vi "Field Add Test Step Field.vi"(6 "nDataType":T1, 7 "sDisplayName":string, 8 "sUnits":string, 9 "sValue":string, 10 "sxFieldId":string, 11 "Fields In":T2[](array[typedef])) -> (3 "Fields Out":T2[](array[typedef]))   [LabVIEW 2011]
uses:
  Field Record.ctl
  Field DataTypes.ctl
  Field NextItem.ctl
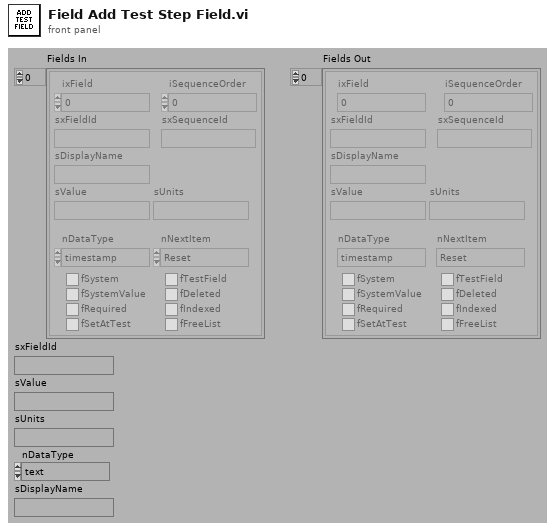
[diagram p1: front panel]
types:
  T1 = typedef "Field DataTypes.ctl" = enum32{"text", "numeric", "list", "timestamp", "boolean"}
  T2 = typedef "Field Record.ctl" = cluster{"ixField":i32, "iSequenceOrder":i32, "sxFieldId":string, "sxSequenceId":string, "sDisplayName":string, "sValue":string, "sUnits":string, "nDataType":T1, "nNextItem":T3, "fSystem":bool, "fSystemValue":bool, "fRequired":bool, "fSetAtTest":bool, "fTestField":bool, "fDeleted":bool, "fIndexed":bool, "fFreeList":bool}
  T3 = typedef "Field NextItem.ctl" = enum32{"Reset", "Retain", "Auto-Increment"}
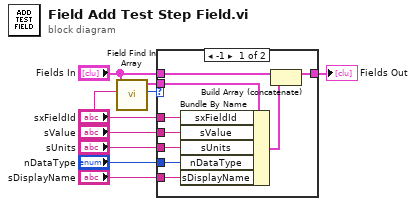
[diagram p0: block diagram]
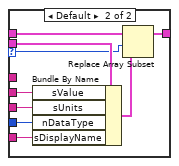
[diagram p2: hidden frame]
diagram:
  n1 = call "Field Find In Array.vi"("FieldID or Display Name(\"\")"="sxFieldId", "Field Array"="Fields In") -> ("Index"=w5:i32, "Field"=w9:T2)  [unwired: 1 in, 7 out]
  n2 = case shown="-1" w5 {
    selector: w5 -> [_ w23]
    tunnel: w9 -> [w17 w27]
    tunnel: "Fields In" -> [w18 w26]
    tunnel: [w16 w22] -> w7
    tunnel: "sValue" -> [w13 w25]
    tunnel: "sxFieldId" -> [w15 _]
    tunnel: "sUnits" -> [w12 w21]
    tunnel: "nDataType" -> [w11 w20]
    tunnel: "sDisplayName" -> [w10 w19]
    frame -1 {
      n3 = Bundle By Name(cluster=w17, "sxFieldId"=w15, "sValue"=w13, "sUnits"=w12, "nDataType"=w11, "sDisplayName"=w10) -> (w14:T2)
      n4 = Build Array (concatenate)(w18, w14) -> (w16:T2[])
    }
    frame Default {
      n5 = Bundle By Name(cluster=w27, "sValue"=w25, "sUnits"=w21, "nDataType"=w20, "sDisplayName"=w19) -> (w24:T2)
      n6 = Replace Array Subset(array=w26, new element=w24, index=w23) -> (w22:T2[])
    }
  }
  "Fields Out" <- w7
